vi "GetDiagramInputs.vi"(6 "error in":errorcluster, 9 "Loop in":refnum<class "Loop.lvclass">) -> (0 "error out":errorcluster, 3 "Loop out":refnum<class "Loop.lvclass">, 4 "inputs terminals":refnum<class "Terminal.lvclass">[][](array[class]))   [LabVIEW 2014, in "Loop.lvclass"]
uses:
  Loop.lvclass
  Terminal/Terminal.lvclass
  Loop.lvclass/Loop.ctl
  ShiftRegister/ShiftRegister.lvclass/ShiftRegister.ctl
  Tunnel/Tunnel.lvclass/Tunnel.ctl
  Structure/Structure.lvclass
  ShiftRegister/ShiftRegister.lvclass
  Tunnel/Tunnel.lvclass
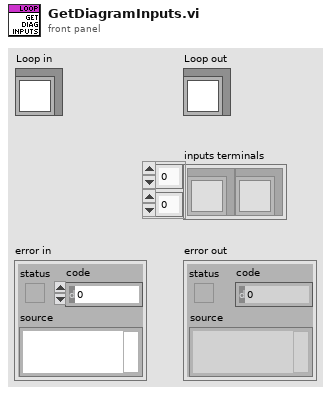
[diagram p1: front panel]
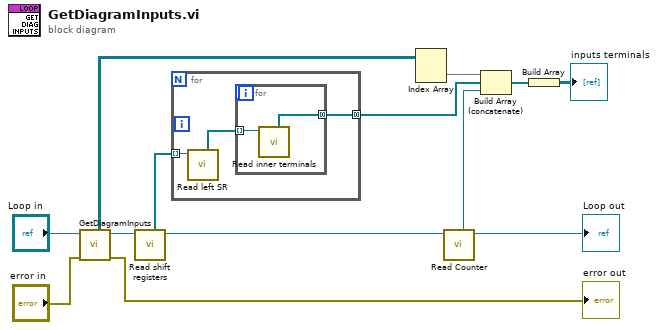
[diagram p0: block diagram]
diagram:
  n1 = call-parent "GetDiagramInputs.vi"("error in"="error in", "Structure in"="Loop in") -> ("error out"=→"error out":errorcluster, "Structure out"=w10:refnum<class "Loop.lvclass">, "inputs terminals"=w6:refnum<class "Terminal.lvclass">[][])  [unwired: 5 in]
  n2 = call "Read shift registers.vi"("Loop in"=w10) -> ("Loop out"=w8:refnum<class "Loop.lvclass">, "shift registers"=w7:refnum<class "ShiftRegister.lvclass">[])  [unwired: 7 in]
  n3 = for {
    tunnel: w7 -> [w16] mode=indexing
    tunnel: [w14] -> w4 mode=concatenating
    n4 = call "Read left SR.vi"("ShiftRegister in"=w16) -> ("left SR"=w15:refnum<class "LeftShiftRegister.lvclass">[])  [unwired: 7 in, 1 out]
    n5 = for {
      tunnel: w15 -> [w18] mode=indexing
      tunnel: [w17] -> w14 mode=concatenating
      n6 = call "Read inner terminals.vi"("Tunnel in"=w18) -> ("inner terminals"=w17:refnum<class "Terminal.lvclass">[])  [unwired: 7 in, 1 out]
    }
  }
  n7 = Index Array(array=w6) -> (element=w5:refnum<class "Terminal.lvclass">[])  [unwired: 2 in]
  n8 = call "Read Counter.vi"("Loop in"=w8) -> ("Loop out"=→"Loop out":refnum<class "Loop.lvclass">, "counter"=w3:refnum<class "Terminal.lvclass">)  [unwired: 7 in]
  n9 = Build Array (concatenate)(w5, w4, w3) -> (w2:refnum<class "Terminal.lvclass">[])
  n10 = Build Array(w2) -> (→"inputs terminals":refnum<class "Terminal.lvclass">[][])
